vi "PUT_item_by_snapshot_id.vi"(9 "Cluster":T1, 10 "SnapID":string, 11 "API Key":string="0") -> (3 "put_in_db_header":string="0\r\nContent-Length: 58\r\nConnection: close\r\n\r\n")   [LabVIEW 2024]
uses:
  <vilib>/httpClient/PUTBuffer.vi
  <vilib>/httpClient/LabVIEWHTTPClient.lvlib
panel:
  out "manipulate_oil_levels":T1
  out "JSON string":string="0"
  out "error out json":errorcluster
  out "body":string="0"
  out "error out put":errorcluster
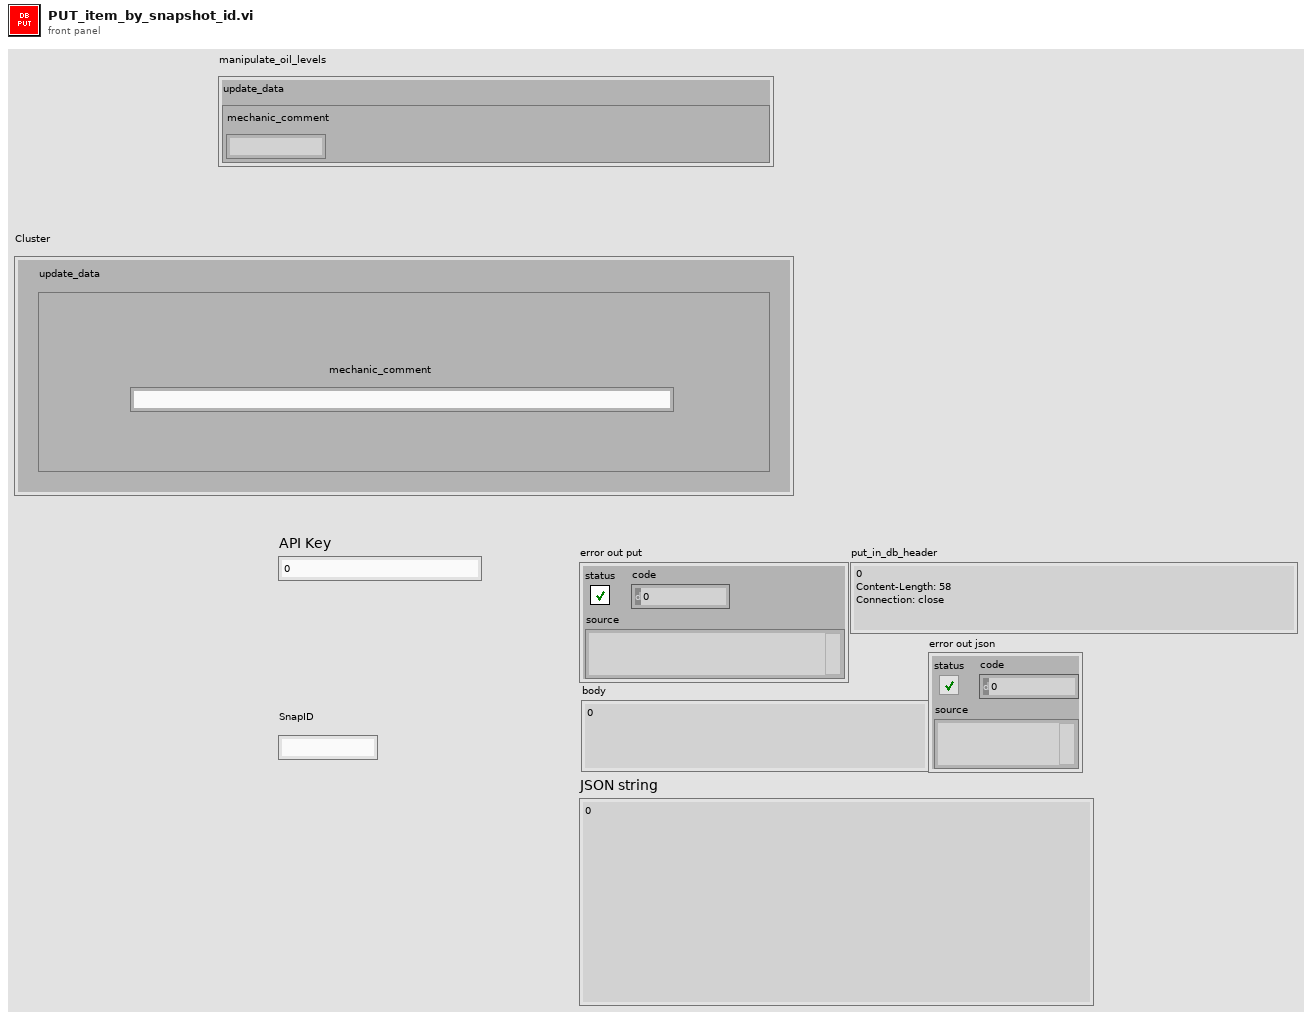
[diagram p1: front panel]
types:
  T1 = cluster{"update_data":cluster{"mechanic_comment":string}}
  T2 = typedef "LabVIEWHTTPClient.lvlib/ClientHandle.ctl" = refnum<k1>
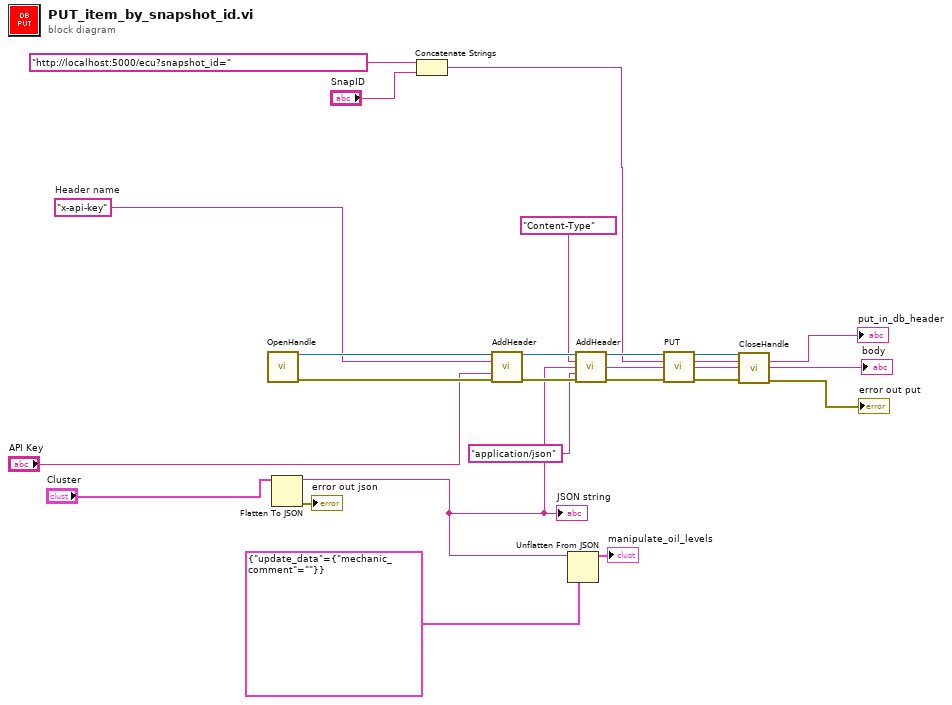
[diagram p0: block diagram]
diagram:
  w16 = "x-api-key"  # Header name
  n1 = call <vilib>:"OpenHandle.vi"() -> ("client handle out"=w17:T2, "error out"=w18:errorcluster)  [unwired: 14 in]
  n2 = Flatten To JSON(anything="Cluster") -> (JSON string=w7:string, 11:→"error out json":errorcluster)  [unwired: 2 in]
  "JSON string" <- w7
  n3 = Concatenate Strings("http://localhost:5000/ecu?snapshot_id=" ("url"), "SnapID") -> (w3:string)
  n4 = call <vilib>:"AddHeader.vi"("client handle"=w17, "header"=w16, "value"="API Key", "error in (no error)"=w18) -> ("client handle out"=w13:T2, "error out"=w10:errorcluster)  [unwired: 10 in]
  n5 = Unflatten From JSON(JSON string=w7, type and defaults=T1 {"update_data"={"mechanic_comment"=""}}) -> (value=→"manipulate_oil_levels":T1)  [unwired: 5 in, 1 out]
  n6 = call <vilib>:"AddHeader.vi"("client handle"=w13, "header"="Content-Type", "value"="application/json", "error in (no error)"=w10) -> ("client handle out"=w12:T2, "error out"=w11:errorcluster)  [unwired: 10 in]
  n7 = call-poly <vilib>:"PUT.vi"("client handle"=w12, "url"=w3, "buffer"=w7, "error in (no error)"=w11) -> ("client handle out"=w20:T2, "headers"=→"put_in_db_header":string, "body"=→"body":string, "error out"=w19:errorcluster)  [unwired: 8 in]
  n8 = call <vilib>:"CloseHandle.vi"("client handle"=w20, "error in (no error)"=w19) -> ("error out"=→"error out put":errorcluster)  [unwired: 13 in]
